vi "Enumerator Current Node.vi"(8 "error in (no error)":errorcluster, 11 "List in":refnum<class "DoublyLinkedList.lvclass">) -> (0 "error out":errorcluster, 2 "Node":refnum<class "DoublyNode.lvclass">, 3 "List out":refnum<class "DoublyLinkedList.lvclass">)   [LabVIEW 2021, in "DoublyLinkedList.lvclass"]
uses:
  DoublyLinkedList.lvclass
  DoublyNode/DoublyNode.lvclass
  DoublyLinkedList.lvclass/DoublyLinkedList.ctl
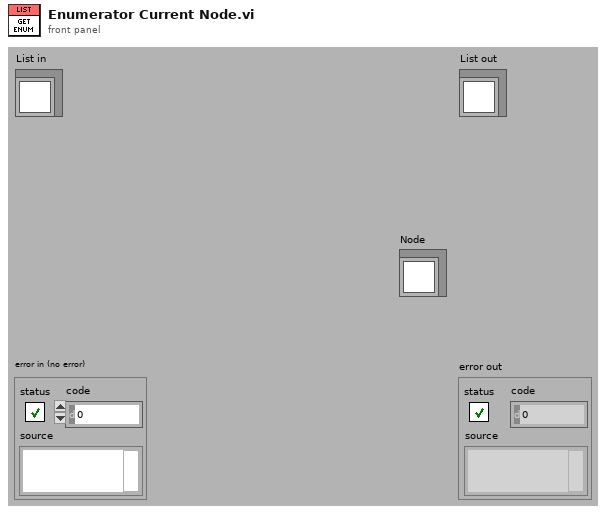
[diagram p1: front panel]
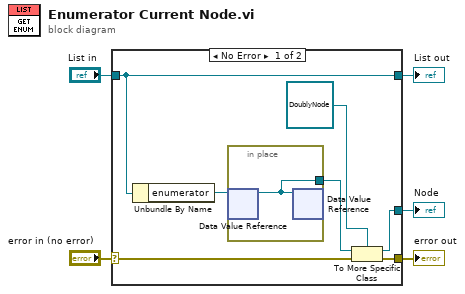
[diagram p0: block diagram]
diagram:
  n1 = case shown="No Error" "error in (no error)" {
    selector: "error in (no error)" -> [w7 w15]
    tunnel: [w6 w15] -> w4
    tunnel: [w12 w14] -> w2
    tunnel: "List in" -> [w12 w14]
    tunnel: [w10 _] -> w1
    frame No Error {
      n2 = Unbundle By Name(w12) -> ("enumerator"=w9:refnum<data-value>)
      n3 = in-place {
        in-place-border: [w13] -> w8
        n4 = in-place-dvr #1(w9) -> (w13:refnum<class "IDoublyNode.lvclass">)  [unwired: 1 out]
        n5 = in-place-dvr #1(w13) -> ()  [unwired: 2 out]
      }
      n6 = To More Specific Class(target class=refnum<class "DoublyNode.lvclass"> refnum ("Node.lvclass"), reference=w8, error in=w7) -> (specific class reference=w10:refnum<class "DoublyNode.lvclass">, error out=w6:errorcluster)
    }
    frame Error {
    }
  }
  "error out" <- w4
  "List out" <- w2
  "Node" <- w1
